vi "Joystick mapping.vi"(11 "JoystickDevRef":T1={"Device"=enum."USB 1"}) -> (2 "Joystick Buttons":T3, 3 "Joystick Axis":T4)   [LabVIEW 2014]
uses:
  Joystick Axis typedefs.ctl
  Joystick Buttons typedef.ctl
  <vilib>/Rock Robotics/WPI/Joystick/WPI_JoystickDevRef.ctl
  <vilib>/Rock Robotics/WPI/Joystick/WPI_JoystickDeviceEnum.ctl
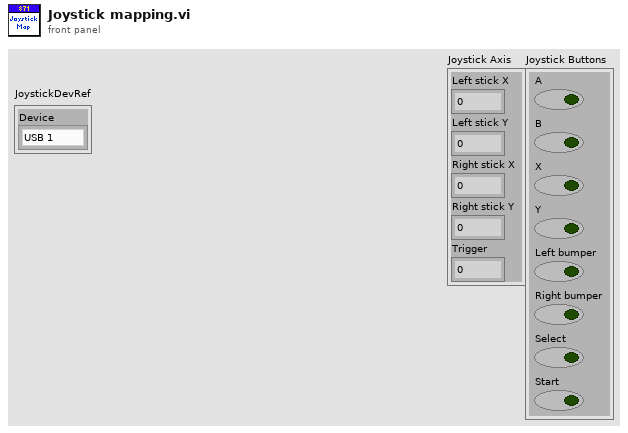
[diagram p1: front panel]
types:
  T1 = typedef "WPI_JoystickDevRef.ctl" = cluster{"Device":T2}
  T2 = typedef "WPI_JoystickDeviceEnum.ctl" = enum16{"USB 0", "USB 1", "USB 2", "USB 3", "USB 4", "USB 5"}
  T3 = typedef "Joystick Buttons typedef.ctl" = cluster{"A":bool, "B":bool, "X":bool, "Y":bool, "Left bumper":bool, "Right bumper":bool, "Select":bool, "Start":bool}
  T4 = typedef "Joystick Axis typedefs.ctl" = cluster{"Left stick X":dbl, "Left stick Y":dbl, "Right stick X ":dbl, "Right stick Y":dbl, "Trigger":dbl}
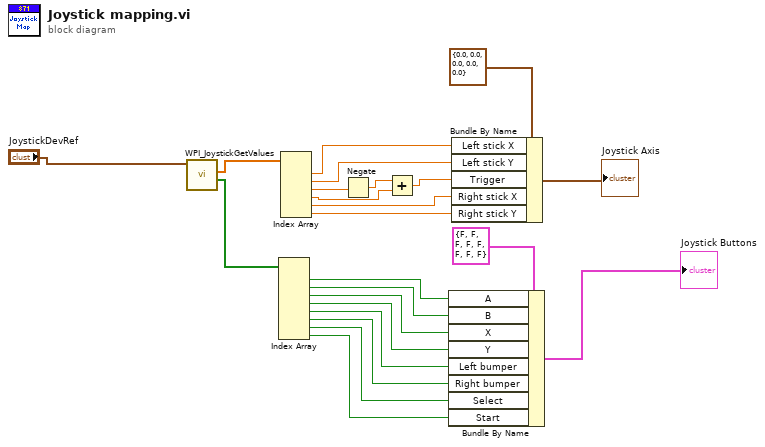
[diagram p0: block diagram]
diagram:
  n1 = call <vilib>:"WPI_JoystickGetValues.vi"("JoystickDevRef"="JoystickDevRef") -> ("Buttons"=w13:bool[], "Axes"=w23:dbl[])  [unwired: 6 in, 3 out]
  n2 = Index Array(array=w13) -> (element #1=w9:bool, element #2=w8:bool, element #3=w7:bool, element #4=w6:bool, element #5=w5:bool, element #6=w4:bool, element #7=w3:bool, element #8=w2:bool)  [unwired: 8 in]
  n3 = Index Array(array=w23) -> (element #1=w21:dbl, element #2=w20:dbl, element #3=w19:dbl, element #4=w17:dbl, element #5=w15:dbl, element #6=w14:dbl)  [unwired: 6 in]
  n4 = Negate(x=w19) -> (-x=w18:dbl)
  n5 = Add(x=w18, y=w17) -> (x+y=w16:dbl)
  n6 = Bundle By Name(cluster=T3 {"A"=FALSE, "B"=FALSE, "X"=FALSE, "Y"=FALSE, "Left bumper"=FALSE, "Right bumper"=FALSE, "Select"=FALSE, "Start"=FALSE} ("Joystick Buttons"), "A"=w9, "B"=w8, "X"=w7, "Y"=w6, "Left bumper"=w5, "Right bumper"=w4, "Select"=w3, "Start"=w2) -> (→"Joystick Buttons":T3)
  n7 = Bundle By Name(cluster=T4 {"Left stick X"=0.0, "Left stick Y"=0.0, "Right stick X "=0.0, "Right stick Y"=0.0, "Trigger"=0.0} ("Joystick Axis"), "Left stick X"=w21, "Left stick Y"=w20, "Trigger"=w16, "Right stick X"=w15, "Right stick Y"=w14) -> (→"Joystick Axis":T4)
